vi "AVI Load.vi"() -> ()   [LabVIEW 2017]
panel:
  in  "Intensity":cluster{i16, i16}(slide)={0, 4095} scale=0.0..4095.0
  in  "Play":bool
  in  "Slide":i32(slide) scale=1.0..2096.0
  out "Numeric":u32
  out "Image":T1(plugin-control)
  in  "AVI File Path":path
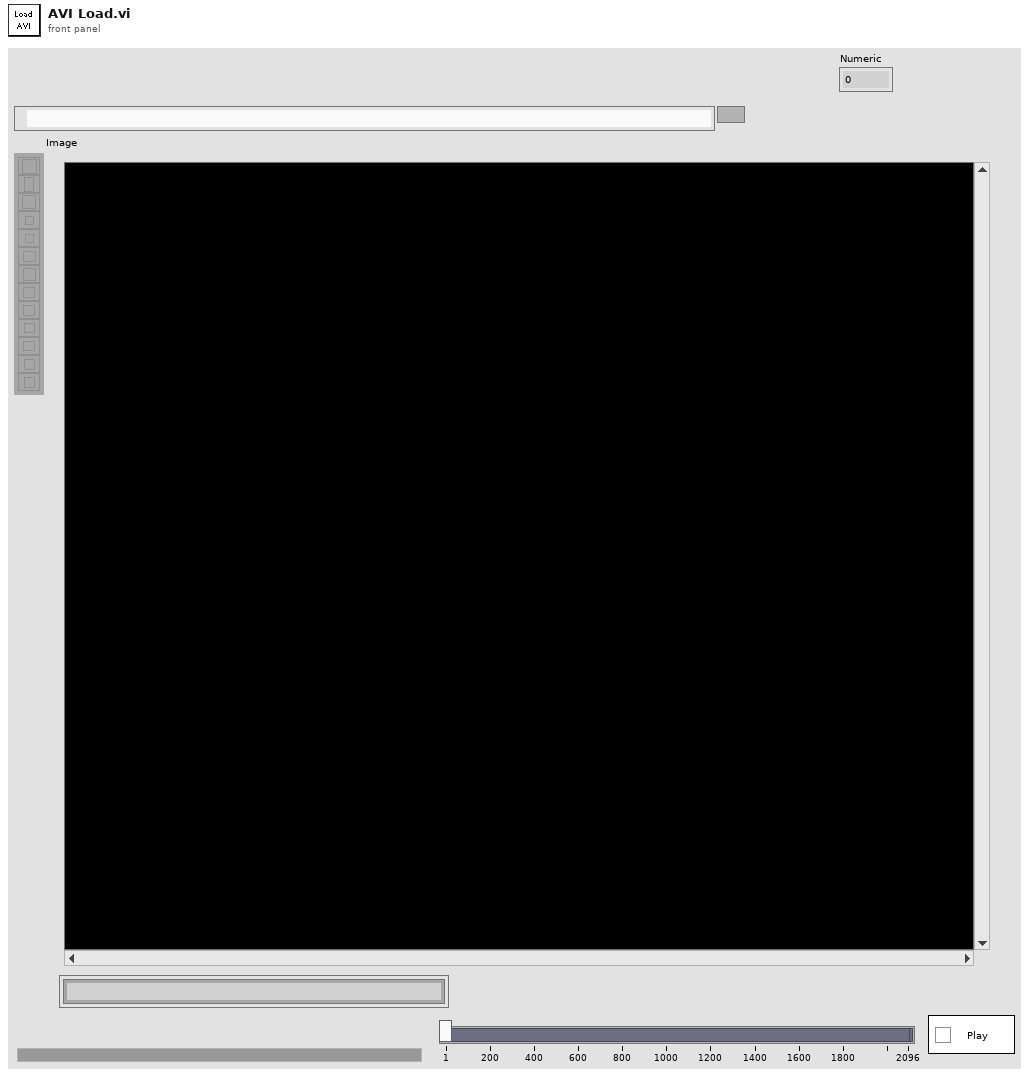
[diagram p1: front panel]
types:
  T1 = typedef "IMAQ Image.ctl" = refnum<image>
  T2 = typedef "Image Type" = u32
  T3 = typedef "IMAQ AVI2 Refnum.ctl" = refnum<k20>
  T4 = cluster{"Conversion Method":u32, "Minimum Value":i32, "Maximum Value":i32, "Number Of Shifts":i32}
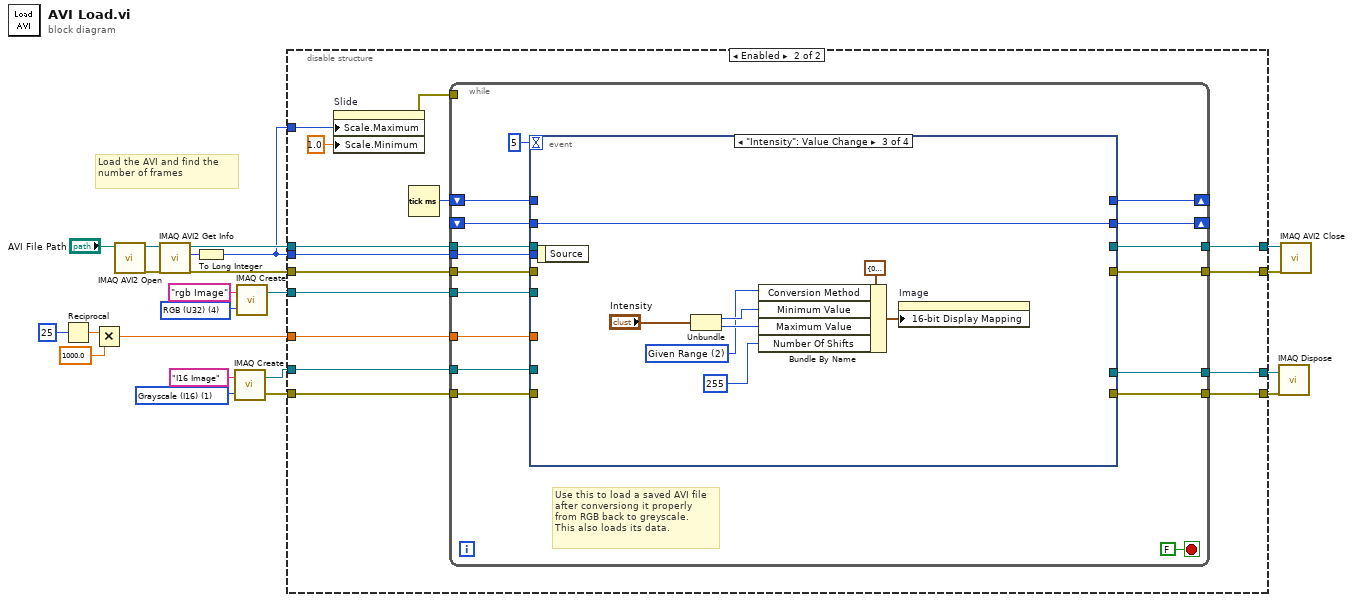
[diagram p0: block diagram]
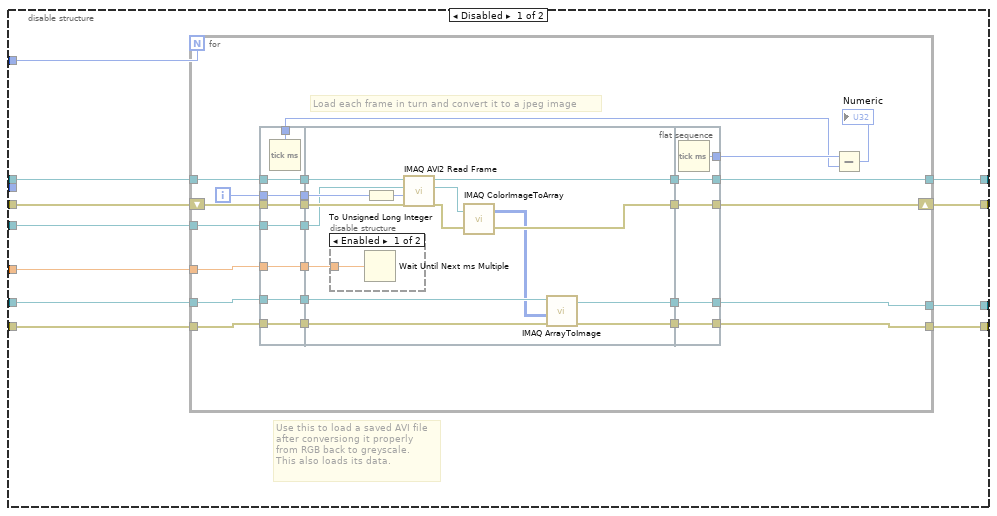
[diagram p2: hidden frame]
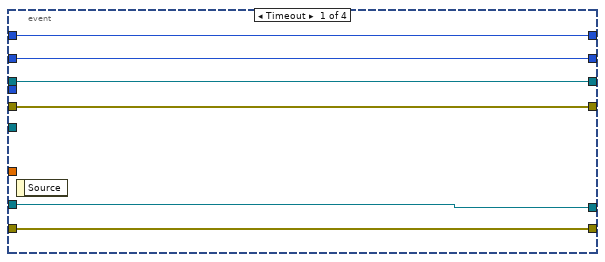
[diagram p4: hidden frame]
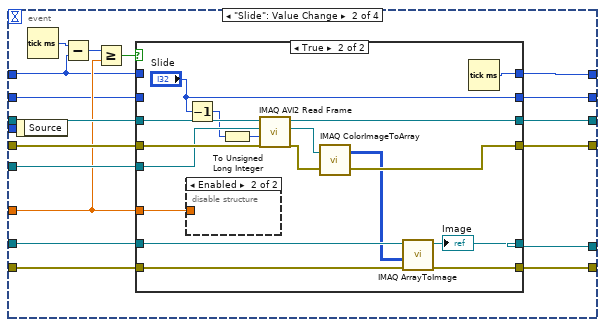
[diagram p5: hidden frame]
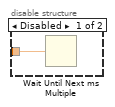
[diagram p7: hidden frame]
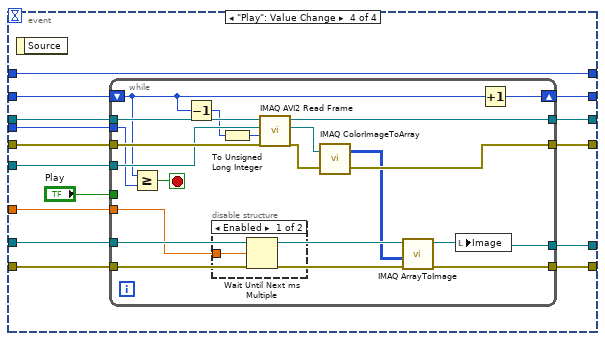
[diagram p8: hidden frame]
diagram:
  w11 = T2 1 items=["Grayscale (U8)", "Grayscale (I16)", "Grayscale (SGL)", "Complex (CSG)", "RGB (U32)", "HSL (U32)", "RGB (U64)", "Grayscale (U16)"] ("Image Type")
  w13 = T2 4 items=["Grayscale (U8)", "Grayscale (I16)", "Grayscale (SGL)", "Complex (CSG)", "RGB (U32)", "HSL (U32)", "RGB (U64)", "Grayscale (U16)"] ("Image Type")
  # "Load the AVI and find the number of frames"
  n1 = Reciprocal(x=25) -> (1/x=w4:dbl)
  n2 = Multiply(x=w4, y=1000.0) -> (x*y=w2:dbl)
  n3 = call "IMAQ AVI2 Open"("AVI File Path"="AVI File Path") -> ("error out"=w22:errorcluster, "AVI Refnum"=w21:T3)  [unwired: 9 in]
  n4 = call "IMAQ AVI2 Get Info"("error in (no error)"=w22, "AVI Refnum"=w21) -> ("error out"=w19:errorcluster, "Number of Frames"=w20:u32, "AVI Refnum (duplicate)"=w18:T3)  [unwired: 5 in, 2 out]
  n5 = To Long Integer(number=w20) -> (32bit integer=w1:i32)
  n6 = call "IMAQ Create"("Image Name"="I16 Image", "Image Type"=w11) -> ("New Image"=w9:T1, "error out"=w8:errorcluster)  [unwired: 2 in, 1 out]
  n7 = call "IMAQ Create"("Image Name"="rgb Image", "Image Type"=w13) -> ("New Image"=w12:T1)  [unwired: 2 in, 2 out]
  n8 = disable-structure shown="Enabled" {
    disable-tunnel: w19 -> [w33 w102]
    disable-tunnel: w1 -> [w32 w91]
    disable-tunnel: w18 -> [w31 w101]
    disable-tunnel: [w30 w100] -> w17
    disable-tunnel: [w29 w99] -> w16
    disable-tunnel: w12 -> [w28 w98]
    disable-tunnel: w9 -> [w27 w97]
    disable-tunnel: w8 -> [w26 w96]
    disable-tunnel: [w25 w95] -> w7
    disable-tunnel: [w24 w94] -> w6
    disable-tunnel: w2 -> [w23 w93]
    disable-tunnel: w1 -> [_ w88]
    frame Disabled {
      # "Use this to load a saved AVI file\nafter conversiong it properly\nfrom RGB back to greyscale.\nThis also loads its data."
      n9 = for {
        N: w32 -> [_]
        tunnel: [w55] -> w30
        tunnel: w31 -> [w56]
        shift-right: [w57] -> w29
        shift-left: w33 -> [w54]
        tunnel: w28 -> [w53]
        tunnel: w27 -> [w52]
        tunnel: w26 -> [w51]
        tunnel: [w50] -> w24
        tunnel: [w49] -> w25
        tunnel: w23 -> [w48]
        i -> [w58]
        # "Load each frame in turn and convert it to a jpeg image"
        n10 = flat-sequence {
          tunnel: w48 -> [w60]
          tunnel: w51 -> [w61]
          tunnel: w52 -> [w62]
          tunnel: w53 -> [w63]
          tunnel: w54 -> [w64]
          tunnel: w56 -> [w65]
          tunnel: w58 -> [w66]
          tunnel: [w66] -> w47
          tunnel: [w65] -> w46
          tunnel: [w64] -> w45
          tunnel: [w63] -> w44
          tunnel: [w62] -> w43
          tunnel: [w61] -> w42
          tunnel: [w60] -> w41
          tunnel: [w59] -> w35
          tunnel: w47 -> [w81]
          tunnel: w46 -> [w79]
          tunnel: w45 -> [w76]
          tunnel: w44 -> [w74]
          tunnel: w43 -> [w72]
          tunnel: w42 -> [w71]
          tunnel: w41 -> [w67]
          tunnel: [w80] -> w40
          tunnel: [w78] -> w39
          tunnel: [w69] -> w38
          tunnel: [w68] -> w37
          tunnel: [w84] -> w49
          tunnel: [w85] -> w50
          tunnel: [w86] -> w55
          tunnel: [w87] -> w57
          tunnel: w40 -> [w87]
          tunnel: w39 -> [w86]
          tunnel: w38 -> [w85]
          tunnel: w37 -> [w84]
          tunnel: [w83] -> w36
          frame #0 {
            n11 = Tick Count (ms)() -> (millisecond timer value=w59:u32)
          }
          frame #1 {
            n12 = disable-structure shown="Enabled" {
              disable-tunnel: w67 -> [w82 _]
              frame Enabled {
                n13 = Wait Until Next ms Multiple(millisecond multiple=w82) -> ()  [unwired: 1 out]
              }
              frame Disabled {
              }
            }
            n14 = To Unsigned Long Integer(number=w81) -> (unsigned 32bit integer=w75:u32)
            n15 = call "IMAQ AVI2 Read Frame"("error in (no error)"=w76, "Frame Number"=w75, "Image"=w74, "AVI Refnum"=w79) -> ("error out"=w77:errorcluster, "Image Out"=w73:T1, "AVI Refnum (duplicate)"=w78:T3)  [unwired: 5 in]
            n16 = call "IMAQ ColorImageToArray"("Image"=w73, "error in (no error)"=w77) -> ("Image Pixels (U32)"=w70:u32[][], "error out"=w80:errorcluster)  [unwired: 1 in, 2 out]
            n17 = call "IMAQ ArrayToImage"("error in (no error)"=w71, "Image Pixels (I16)"=w70, "Image"=w72) -> ("error out"=w69:errorcluster, "Image Out"=w68:T1)  [unwired: 7 in]
          }
          frame #2 {
            n18 = Tick Count (ms)() -> (millisecond timer value=w83:u32)
          }
        }
        n19 = Subtract(x=w36, y=w35) -> (x-y=→"Numeric":u32)
      }
    }
    frame Enabled {
      n20 = property on="Slide" class="Slide (strict)"("Scale.Maximum"=w91, "Scale.Minimum"=1.0 ("Scale.Range:Minimum")) -> (error out=w90:errorcluster)  [unwired: 2 in, 1 out]
      n21 = Tick Count (ms)() -> (millisecond timer value=w89:u32)
      n22 = while {
        tunnel: w102 -> [w119]
        tunnel: w101 -> [w118]
        tunnel: [w117] -> w100
        tunnel: [w116] -> w99
        tunnel: w98 -> [w115]
        tunnel: w97 -> [w114]
        tunnel: w96 -> [w113]
        tunnel: [w112] -> w95
        tunnel: [w111] -> w94
        tunnel: w93 -> [w110]
        tunnel: w90 -> [_]
        shift-right: [w107] -> _
        shift-left: w89 -> [w106]
        shift-right: [w105] -> _
        shift-left: _ -> [w104]
        tunnel: w88 -> [w103]
        stop <- FALSE stop-if-true
        # "Use this to load a saved AVI file\nafter conversiong it properly\nfrom RGB back to greyscale.\nThis also loads its data."
        n23 = event shown="[2] \"Intensity\": Value Change" {
          selector: _ -> [_ _ _ _]
          dyn-events: _ -> [_ _ _ _]
          timeout: 5 -> [_ _ _ _]
          tunnel: w119 -> [w124 w141 _ w188]
          tunnel: w118 -> [w125 w142 _ w189]
          tunnel: [w125 w136 _ w183] -> w117
          tunnel: [w124 w135 _ w182] -> w116
          tunnel: w115 -> [_ w140 _ w187]
          tunnel: w114 -> [w123 w139 _ w186]
          tunnel: w113 -> [w122 w138 _ w185]
          tunnel: [w123 w134 _ w181] -> w112
          tunnel: [w122 w137 _ w184] -> w111
          tunnel: w110 -> [_ w131 _ w180]
          tunnel: [w121 w129 _ w179] -> w107
          tunnel: w106 -> [w121 w128 _ w179]
          tunnel: [w120 w127 w174 w178] -> w105
          tunnel: w104 -> [w120 w126 w174 w177]
          tunnel: w103 -> [_ _ _ w176]
          event Timeout {
            n24 = event-data() -> ()  [unwired: 1 in, 1 out]
          }
          event "Slide": Value Change {
            n25 = event-data() -> ()  [unwired: 1 in, 1 out]
            n26 = Tick Count (ms)() -> (millisecond timer value=w133:u32)
            n27 = Subtract(x=w133, y=w128) -> (x-y=w132:u32)
            n28 = Greater Or Equal?(x=w132, y=w131) -> (x >= y?=w130:bool)
            n29 = case shown="True" w130 {
              tunnel: w142 -> [w148 w165]
              tunnel: w141 -> [w147 w164]
              tunnel: w140 -> [_ w163]
              tunnel: w131 -> [_ w162]
              tunnel: w139 -> [w146 w161]
              tunnel: w138 -> [w145 w160]
              tunnel: [w145 w159] -> w137
              tunnel: [w148 w158] -> w136
              tunnel: [w147 w157] -> w135
              tunnel: [w146 w149] -> w134
              tunnel: [w144 w151] -> w129
              tunnel: w128 -> [w144 _]
              tunnel: [w143 "Slide"] -> w127
              tunnel: w126 -> [w143 _]
              frame False {
              }
              frame True {
                n30 = Decrement(x="Slide") -> (x-1=w152:i32)
                n31 = disable-structure shown="Enabled" {
                  disable-tunnel: w162 -> [w166 _]
                  frame Disabled {
                    n32 = Wait Until Next ms Multiple(millisecond multiple=w166) -> ()  [unwired: 1 out]
                  }
                  frame Enabled {
                  }
                }
                n33 = To Unsigned Long Integer(number=w152) -> (unsigned 32bit integer=w155:u32)
                n34 = call "IMAQ AVI2 Read Frame"("error in (no error)"=w164, "Frame Number"=w155, "Image"=w163, "AVI Refnum"=w165) -> ("error out"=w156:errorcluster, "Image Out"=w154:T1, "AVI Refnum (duplicate)"=w158:T3)  [unwired: 5 in]
                n35 = call "IMAQ ColorImageToArray"("Image"=w154, "error in (no error)"=w156) -> ("Image Pixels (U32)"=w153:u32[][], "error out"=w157:errorcluster)  [unwired: 1 in, 2 out]
                n36 = call "IMAQ ArrayToImage"("error in (no error)"=w160, "Image Pixels (I16)"=w153, "Image"=w161) -> ("error out"=w159:errorcluster, "Image Out"=w149:T1)  [unwired: 7 in]
                "Image" <- w149
                n37 = Tick Count (ms)() -> (millisecond timer value=w151:u32)
              }
            }
          }
          event "Intensity": Value Change {
            w167 = u32 2 items=["Full Dynamic", "Downshift", "Given Range", "90% Dynamic", "Given Percent Range"] ("16-bit Display Mapping:Conversion Method")
            n38 = event-data() -> ()  [unwired: 1 in, 1 out]
            n39 = Unbundle("Intensity") -> (w169:i16, w168:i16)
            n40 = Bundle By Name(cluster=T4 {"Conversion Method"=0, "Minimum Value"=0, "Maximum Value"=0, "Number Of Shifts"=0} ("16-bit Display Mapping:All Elements"), "Conversion Method"=w167, "Minimum Value"=w169, "Maximum Value"=w168, "Number Of Shifts"=255) -> (w171:T4)
            n41 = property on="Image" class="ImageControl"("16-bit Display Mapping"=w171) -> ()  [unwired: 2 in, 2 out]
          }
          event "Play": Value Change {
            n42 = event-data() -> ()  [unwired: 1 in, 1 out]
            n43 = while {
              tunnel: w189 -> [w208]
              tunnel: w188 -> [w207]
              tunnel: w187 -> [w206]
              tunnel: w186 -> [w205]
              tunnel: w185 -> [w204]
              tunnel: [w203] -> w184
              tunnel: [w202] -> w183
              tunnel: [w201] -> w182
              tunnel: [w200] -> w181
              tunnel: w180 -> [w199]
              tunnel: w176 -> [w191]
              tunnel: "Play" -> [_]
              shift-right: [w193] -> w178
              shift-left: w177 -> [w192]
              stop <- w190 stop-if-true
              n44 = Greater Or Equal?(x=w192, y=w191) -> (x >= y?=w190:bool)
              n45 = Decrement(x=w192) -> (x-1=w194:i32)
              n46 = disable-structure shown="Enabled" {
                disable-tunnel: w199 -> [w209 _]
                frame Enabled {
                  n47 = Wait Until Next ms Multiple(millisecond multiple=w209) -> ()  [unwired: 1 out]
                }
                frame Disabled {
                }
              }
              n48 = To Unsigned Long Integer(number=w194) -> (unsigned 32bit integer=w197:u32)
              n49 = call "IMAQ AVI2 Read Frame"("error in (no error)"=w207, "Frame Number"=w197, "Image"=w206, "AVI Refnum"=w208) -> ("error out"=w198:errorcluster, "Image Out"=w196:T1, "AVI Refnum (duplicate)"=w202:T3)  [unwired: 5 in]
              n50 = call "IMAQ ColorImageToArray"("Image"=w196, "error in (no error)"=w198) -> ("Image Pixels (U32)"=w195:u32[][], "error out"=w201:errorcluster)  [unwired: 1 in, 2 out]
              n51 = call "IMAQ ArrayToImage"("error in (no error)"=w204, "Image Pixels (I16)"=w195, "Image"=w205) -> ("error out"=w203:errorcluster, "Image Out"=w200:T1)  [unwired: 7 in]
              n52 = local write "Image"(w200) -> ()
              n53 = Increment(x=w192) -> (x+1=w193:i32)
            }
          }
        }
      }
    }
  }
  n54 = call "IMAQ Dispose"("Image"=w7, "error in (no error)"=w6) -> ()  [unwired: 4 in, 1 out]
  n55 = call "IMAQ AVI2 Close"("error in (no error)"=w16, "AVI Refnum"=w17) -> ()  [unwired: 9 in, 1 out]
